vi "Create_Object.vi"(8 "error in (no error)":errorcluster, 9 "Terminal Map in":map{string, T1}(c390), 10 "owner refnum":variant, 11 "GrowableFunction in":refnum<class "GrowableFunction.lvclass">) -> (0 "error out":errorcluster, 1 "Terminal Map Out":map{string, T1}(c390), 3 "GrowableFunction out":refnum<class "GrowableFunction.lvclass">)   [LabVIEW 2025, in "GrowableFunction.lvclass"]
uses:
  GrowableFunction.lvclass
  C:/Users/mrjak/Documents/GitHub/LVGPT/LabVIEW/VIs/Classes/Node/Node.lvclass
  Terminal.ctl
  Node.lvclass/Node.ctl
  Node.lvclass
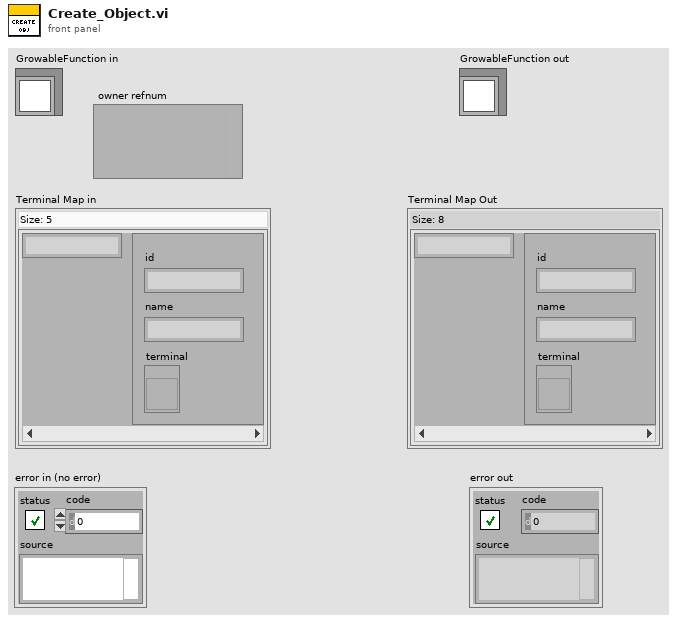
[diagram p1: front panel]
types:
  T1 = typedef "Terminal.ctl" = cluster{"id":string, "name":string, "terminal":refnum<vi>}
  T2 = typedef "LVPointTypeDef.ctl" = cluster{"Horizontal":i16, "Vertical":i16}
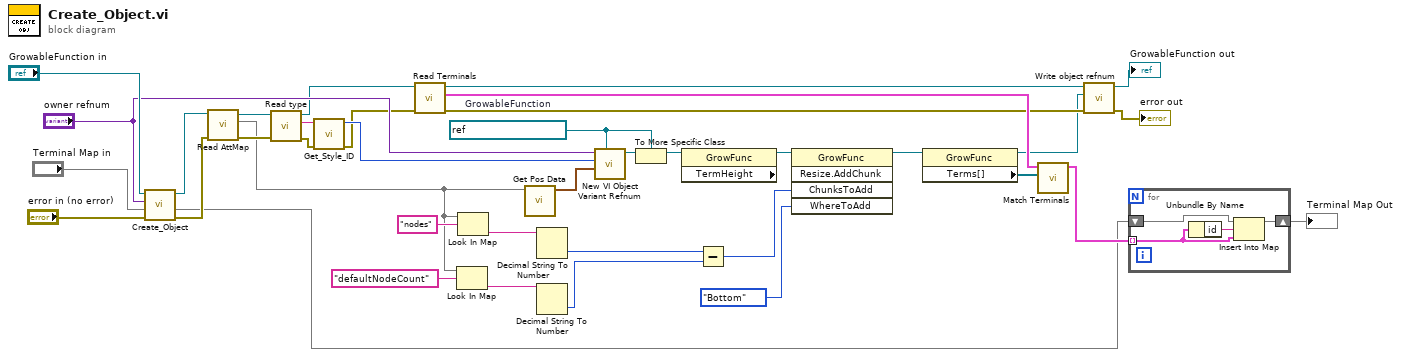
[diagram p0: block diagram]
diagram:
  w25 = refnum<vi> refnum  # GrowableFunction
  n1 = call-parent "Create_Object.vi"("error in (no error)"="error in (no error)", "Terminal Map in"="Terminal Map in", "owner refnum"="owner refnum", "Node in"="GrowableFunction in") -> ("error out"=w23:errorcluster, "Terminal Map Out"=w12:map{string, T1}, "Node out"=w24:refnum<class "GrowableFunction.lvclass">)  [unwired: 5 in]
  n2 = call "Read AttMap.vi"("error in (no error)"=w23, "Node in"=w24) -> ("error out"=w21:errorcluster, "AttMap"=w3:map{string, string}, "Node out"=w20:refnum<class "GrowableFunction.lvclass">)  [unwired: 7 in]
  n3 = call "Read type.vi"("error in (no error)"=w21, "Node in"=w20) -> ("error out"=w17:errorcluster, "type"=w22:string, "Node out"=w15:refnum<class "GrowableFunction.lvclass">)  [unwired: 7 in]
  n4 = call "Get_Style_ID.vi"("error in (no error)"=w17, "Style"=w22) -> ("error out"=w16:errorcluster, "style"=w19:i32)  [unwired: 7 in, 1 out]
  n5 = call "Read Terminals.vi"("error in (no error)"=w16, "Node in"=w15) -> ("error out"=w9:errorcluster, "Terminals"=w14:T1[], "Node out"=w10:refnum<class "GrowableFunction.lvclass">)  [unwired: 7 in]
  n6 = Look In Map(map=w3, key="defaultNodeCount") -> (value=w2:string)  [unwired: 1 in, 1 out]
  n7 = Look In Map(map=w3, key="nodes") -> (value=w32:string)  [unwired: 1 in, 1 out]
  n8 = call "Get Pos Data.vi"("AttMap"=w3) -> ("Position"=w35:T2)  [unwired: 10 in]
  n9 = Decimal String To Number(string=w32) -> (number=w28:i32)  [unwired: 2 in, 1 out]
  n10 = Decimal String To Number(string=w2) -> (number=w1:i32)  [unwired: 2 in, 1 out]
  n11 = call "New VI Object Variant Refnum.vi"("vi object class"=w25, "location"=w35, "style"=w19, "owner refnum"="owner refnum") -> ("object refnum"=w31:refnum<vi>)  [unwired: 6 in, 1 out]
  n12 = To More Specific Class(target class=w25, reference=w31) -> (specific class reference=w26:refnum<vi>)  [unwired: 1 in, 1 out]
  n13 = property class="GrowFunc" props=["TermHeight"](reference=w26) -> (reference out=w5:refnum<vi>)  [unwired: 1 in, 2 out]
  n14 = Subtract(x=w28, y=w1) -> (x-y=w27:i32)
  n15 = invoke class="GrowFunc" method="Resize.AddChunk"(reference=w5, "ChunksToAdd"=w27, "WhereToAdd"=enum8{"Bottom", "Top"}."Bottom" ("Where To Add")) -> (reference out=w30:refnum<vi>)  [unwired: 2 in, 4 out]
  n16 = property class="GrowFunc"(reference=w30) -> (reference out=w8:refnum<vi>, "Terms[]"=w33:refnum<vi>[])  [unwired: 1 in, 1 out]
  n17 = call "Match Terminals.vi"("Terms[]"=w33, "Terminals"=w14) -> ("Terminals Out"=w13:T1[])  [unwired: 9 in]
  n18 = call-dynamic "Write object refnum.vi"("error in (no error)"=w9, "object refnum"=w8, "Node in"=w10) -> ("error out"=→"error out":errorcluster, "Node out"=→"GrowableFunction out":refnum<class "GrowableFunction.lvclass">)  [unwired: 7 in]
  n19 = for {
    shift-right: [w41] -> w11
    shift-left: w12 -> [w42]
    tunnel: w13 -> [w40] mode=indexing
    n20 = Unbundle By Name(w40) -> ("id"=w39:string)
    n21 = Insert Into Map(map in=w42, key=w39, value=w40) -> (map out=w41:map{string, T1})  [unwired: 2 out]
  }
  "Terminal Map Out" <- w11
